vi "Setup Log.vi"(8 "error in (no error)":errorcluster, 10 "Model in":refnum<class "Model.lvclass">, 11 "Boot Loader in":refnum<class "Boot Loader.lvclass">) -> (0 "error out":errorcluster, 2 "Model out":refnum<class "Model.lvclass">, 3 "Boot Loader out":refnum<class "Boot Loader.lvclass">)   [LabVIEW 2016, in "Boot Loader.lvclass"]
uses:
  Boot Loader.lvclass
  Model/Model.lvclass
  Typedefs/TestLogTypes.ctl
  Test Log/Test Log Factory/OperationsLogFactory.lvclass
  Model/Model.lvclass/Model.ctl
  Typedefs/M1M3SupportEUI_TypeDefs.lvlib
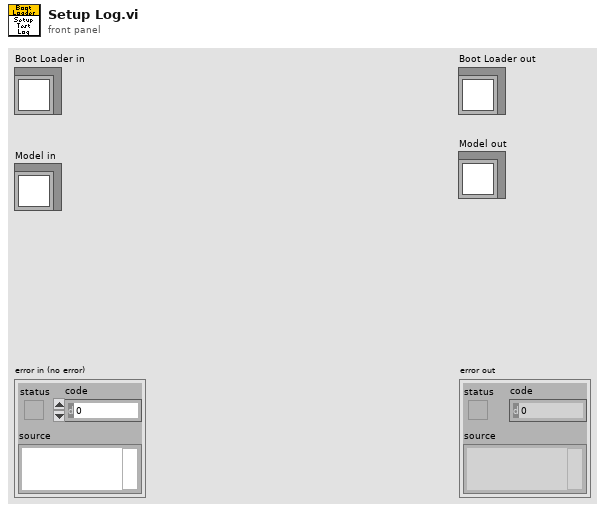
[diagram p1: front panel]
types:
  T1 = typedef "M1M3SupportEUI_TypeDefs.lvlib/TestLogTypes.ctl" = enum16{"CSV Test Log"}
  T2 = typedef "M1M3SupportEUI_TypeDefs.lvlib/TestSettings.ctl" = cluster{"Operator":string}
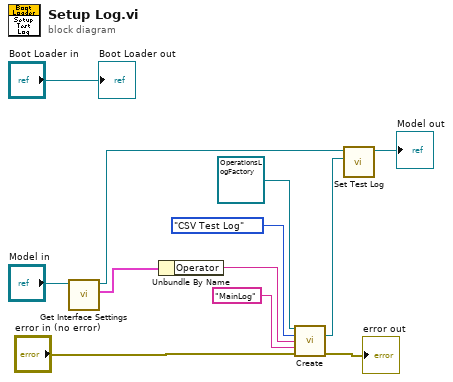
[diagram p0: block diagram]
diagram:
  n1 = call "Get Interface Settings.vi"("Model in"="Model in") -> ("Interface Settings"=w8:T2, "Model out"=w5:refnum<class "Model.lvclass">)  [unwired: 9 in]
  n2 = Unbundle By Name(w8) -> ("Operator"=w2:string)
  n3 = call-dynamic "Create.vi"("Test Log Factory in"=refnum<class "OperationsLogFactory.lvclass"> refnum ("Test Log Factory.lvclass"), "Test Log Types"=TestLogTypes."CSV Test Log" ("TestLogTypes"), "Test Name"=w2, "Scan Name"="MainLog", "error in (no error)"="error in (no error)") -> ("Test Log"=w11:refnum<class "OperationsLog.lvclass">, "error out"=→"error out":errorcluster)  [unwired: 8 in, 1 out]
  n4 = call "Set Test Log.vi"("ITestLog.lvclass"=w11, "Model in"=w5) -> ("Model out"=→"Model out":refnum<class "Model.lvclass">)  [unwired: 9 in]
  "Boot Loader out" <- "Boot Loader in"
